vi "Read Jitter Measurements.vi"(8 "error in (no error)":errorcluster, 9 "Analyzer (0: A0)":i32(ring) items=["A0", "A1"], 10 "Measurement (0: Time Domain Jitter)":i32(ring) items=["Time Domain Jitter", "Frequency Domain Jitter"], 11 "VISA resource name":refnum<visa-resource-name>) -> (0 "error out":errorcluster, 2 "Jitter Measured Value":dbl, 3 "VISA resource name out":refnum<visa-resource-name>)   [LabVIEW 2014, in "Stanford Research SR1.lvlib"]
doc: "Reads the measurement from the Jitter Digital Generator."
uses:
  Stanford Research SR1.lvlib
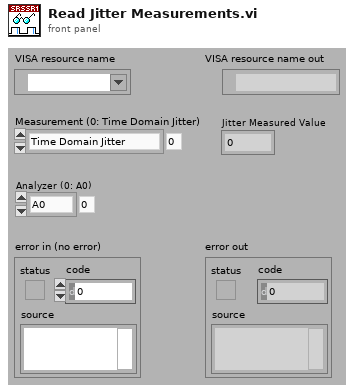
[diagram p1: front panel]
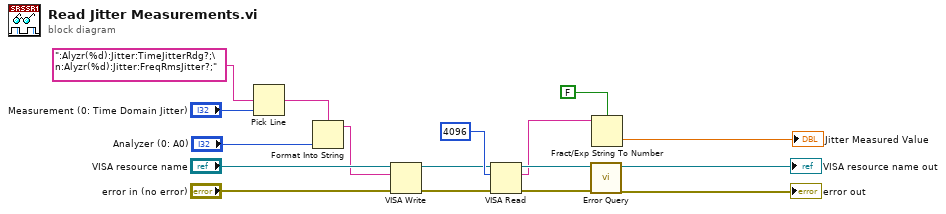
[diagram p0: block diagram]
diagram:
  n1 = Pick Line(multi-line string=":Alyzr(%d):Jitter:TimeJitterRdg?;\n:Alyzr(%d):Jitter:FreqRmsJitter?;", line index="Measurement (0: Time Domain Jitter)") -> (output string=w6:string)  [unwired: 1 in]
  n2 = Format Into String(format string=w6, "Analyzer (0: A0)") -> (resulting string=w4:string)  [unwired: 2 in, 1 out]
  n3 = VISA Write(VISA resource name="VISA resource name", write buffer=w4, error in (no error)="error in (no error)") -> (VISA resource name out=w14:refnum<visa-resource-name>, error out=w13:errorcluster)  [unwired: 1 out]
  n4 = VISA Read(VISA resource name=w14, byte count=u32 4096, error in (no error)=w13) -> (VISA resource name out=w12:refnum<visa-resource-name>, read buffer=w3:string, error out=w11:errorcluster)  [unwired: 1 out]
  n5 = call "Error Query.vi"("error in (no error)"=w11, "VISA resource name"=w12) -> ("error out"=→"error out":errorcluster, "VISA resource name out"=→"VISA resource name out":refnum<visa-resource-name>)  [unwired: 6 in, 2 out]
  n6 = Fract/Exp String To Number(use system decimal point (T)=FALSE, string=w3) -> (number=→"Jitter Measured Value":dbl)  [unwired: 2 in, 1 out]
